vi "Prompt for Step--Init UI.vi"(8 "error in (no error)":errorcluster, 10 "Control Ref Map":map{string, refnum<vi>}(c390), 11 "Step in":refnum<class "Step.lvclass">) -> (0 "error out":errorcluster, 3 "Step out":refnum<class "Step.lvclass">)   [LabVIEW 2020, in "MacroAssert.lvlib" / "Step.lvclass"]
uses:
  Step.lvclass
  Step.lvclass/Step.ctl
  MacroAssert.lvlib
  Support/Get Control Reference by Label (1D STR).vi
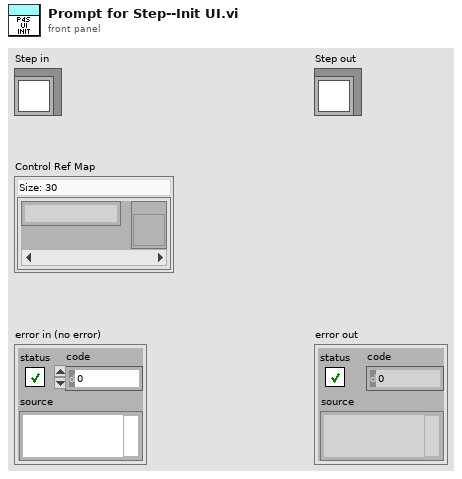
[diagram p1: front panel]
types:
  T1 = typedef "MacroAssert.lvlib/Step Type V3.ctl" = enum16{"Mouse Action", "Keyboard Action", "Window Action", "Timing Action", "Boolean Assertion", "Numeric Assertion", "String Assertion", "Image Assertion"}
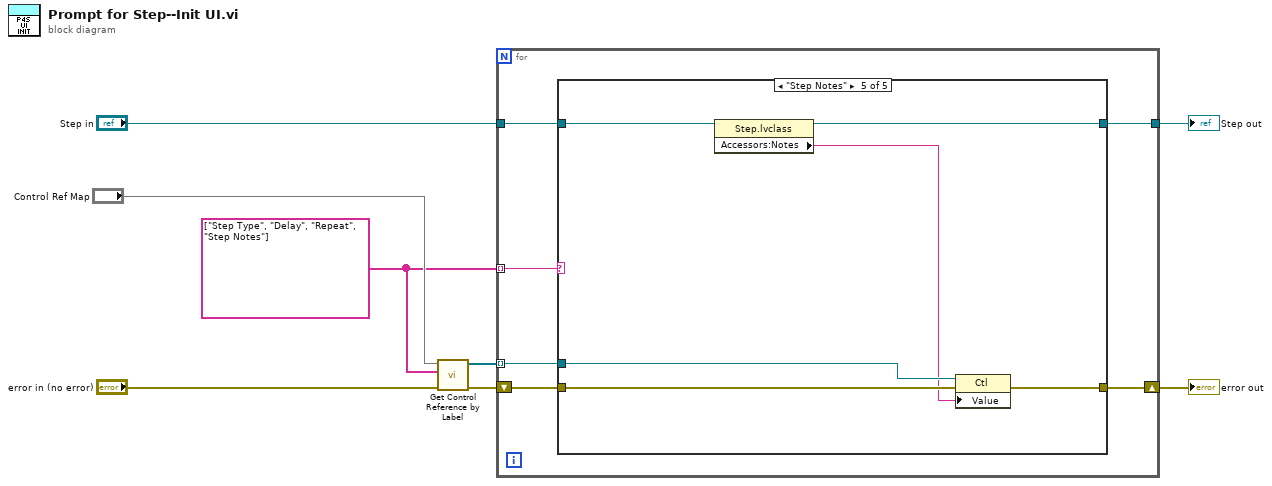
[diagram p0: block diagram]
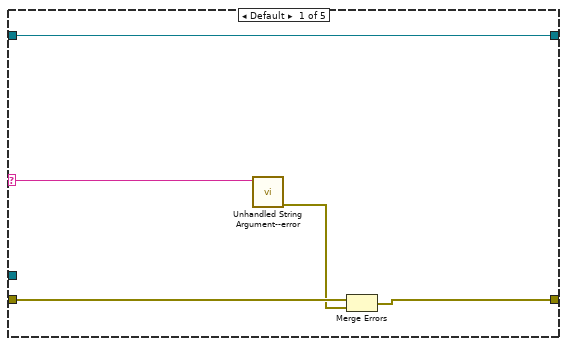
[diagram p2: hidden frame]
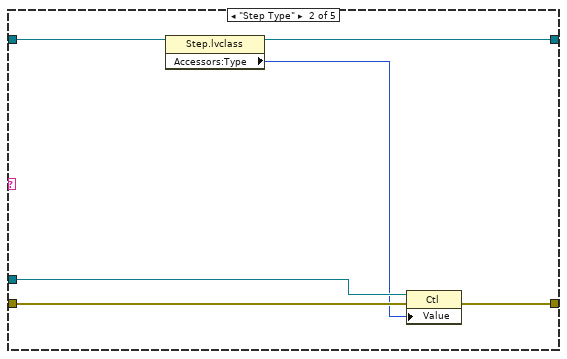
[diagram p3: hidden frame]
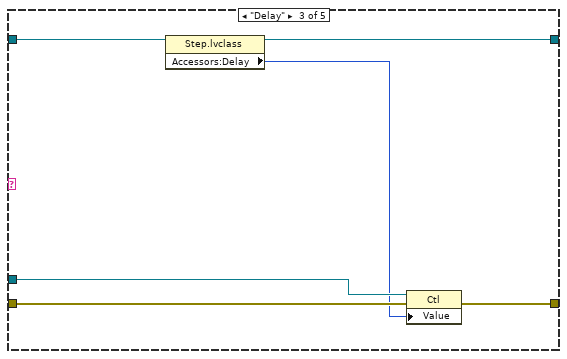
[diagram p4: hidden frame]
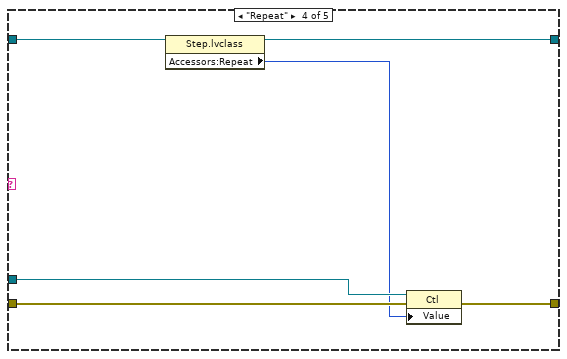
[diagram p5: hidden frame]
diagram:
  w3 = string[] ["Step Type", "Delay", "Repeat", "Step Notes"]
  n1 = call-poly "Get Control Reference by Label.vi"("error in (no error)"="error in (no error)", "Control Names"=w3, "Control Ref Map"="Control Ref Map") -> ("error out"=w5:errorcluster, "Control Refs"=w2:refnum<vi>[])  [unwired: 6 in, 1 out]
  n2 = for {
    tunnel: "Step in" -> [w12]
    tunnel: [w10] -> w7
    tunnel: w3 -> [w13] mode=indexing
    tunnel: w2 -> [w11] mode=indexing
    shift-right: [w9] -> w1
    shift-left: w5 -> [w14]
    n3 = case shown="\"Step Notes\"" w13 {
      selector: w13 -> [w19 _ _ _ _]
      tunnel: w14 -> [w18 w22 w28 w34 w40]
      tunnel: w12 -> [w15 w25 w31 w37 w43]
      tunnel: w11 -> [_ w23 w29 w35 w41]
      tunnel: [w15 w24 w30 w36 w42] -> w10
      tunnel: [w16 w20 w26 w32 w38] -> w9
      frame Default {
        n4 = call "Unhandled String Argument--error.vi"("Argument"=w19) -> ("error out"=w17:errorcluster)  [unwired: 10 in]
        n5 = Merge Errors(w18, w17) -> (w16:errorcluster)
      }
      frame "Step Type" {
        n6 = property class="Step.lvclass"(reference=w25) -> (reference out=w24:refnum<class "Step.lvclass">, "Accessors:Type"=w21:T1)  [unwired: 1 in, 1 out]
        n7 = property class="Ctl"(reference=w23, error in=w22, "Value"=w21) -> (error out=w20:errorcluster)  [unwired: 1 out]
      }
      frame "Delay" {
        n8 = property class="Step.lvclass"(reference=w31) -> (reference out=w30:refnum<class "Step.lvclass">, "Accessors:Delay"=w27:i32)  [unwired: 1 in, 1 out]
        n9 = property class="Ctl"(reference=w29, error in=w28, "Value"=w27) -> (error out=w26:errorcluster)  [unwired: 1 out]
      }
      frame "Repeat" {
        n10 = property class="Step.lvclass"(reference=w37) -> (reference out=w36:refnum<class "Step.lvclass">, "Accessors:Repeat"=w33:i32)  [unwired: 1 in, 1 out]
        n11 = property class="Ctl"(reference=w35, error in=w34, "Value"=w33) -> (error out=w32:errorcluster)  [unwired: 1 out]
      }
      frame "Step Notes" {
        n12 = property class="Step.lvclass"(reference=w43) -> (reference out=w42:refnum<class "Step.lvclass">, "Accessors:Notes"=w39:string)  [unwired: 1 in, 1 out]
        n13 = property class="Ctl"(reference=w41, error in=w40, "Value"=w39) -> (error out=w38:errorcluster)  [unwired: 1 out]
      }
    }
  }
  "error out" <- w1
  "Step out" <- w7
